vi "EOL Sunshade Servo Test.vi"(7 "scaling factor":dbl=11.1, 10 "input cluster":T2={"Application Status"="", "Switch Output Array"=[], "Switch Value Configuration"=[], "NVH Configuration"={"NVH Station?"=FALSE, "nvh app instance path"="", "NVH_ErrorMessages sv url"="", "NVH_Inputs sv url"="", "NVH_MotionNumber sv url"="", "NVH_Outputs sv url"="", "NVH_PartNumber sv url"="", "NVH_PartNumber_Echo sv url"="", "NVH_SerialNumber sv url"="", "NVH_AmbientTempF sv url"=""}, "rs232 port map"={"PMAC"="", "PS Port"="", "LVDT Unit"="", "RS232"=""}, "ethernet address map"={"LVDT 1 Unit"="172.17.53.143", "LVDT Unit 1 port"=0}, "paths"={"Base Path"=path "", "system error log path"=path "", "Error Table Path"=path "C/Labview Code/System/Error Table", "Store errors log path"=path "C/Labview Code/System/Error Table", "data bytes log path"=path "C/Labview Code/System/Error Table", "network path"=path "C/Labview Code/System/Error Table"}, "Station Index"=0, "Store Data"={"Motion Data Array"=[], "Error Table"=[], "Sun Shade Close Force Limits"={"Overall Min"=0.0, "Overall Max"=0.0, "Avg Min"=0.0, "Avg Max"=0.0, "Truncation Start"=0.0, "Truncation End"=0.0, "Variance"=0.0, "Check Noise"=FALSE}, "Sun Shade Open Force Limits"={"Overall Min"=0.0, "Overall Max"=0.0, "Avg Min"=0.0, "Avg Max"=0.0, "Truncation Start"=0.0, "Truncation End"=0.0, "Variance"=0.0, "Check Noise"=FALSE}, "Sunshade Open Data"=[], "Sunshade Close Data"=[], "Module Info"={"Serial Number"="", "Pallet Number"="", "Sunshade Color"="", "Inalfa Part Number"="", "Customer Number"=""}, "Sunsahde Close Raw Data"=[], "Sunshade Open Raw Data"=[], "Software Version"=[], "Constant Version"=[], "Hardware Version"=[], "Inalfa Part Number ECU"=[], "LVDT Data"=[], "Communication Line 1"=[], "Communication Line 2"=[], "Anti Pinch Force"=[], "Cycle Time"="", "Anti Pinch Vent Force"=[], "iGPS LVDT Data"=[], "data bytes log"=""}, "D in map"={"Abort Test"=enum."Dev2/port2/line6", "Start Test"=enum."Dev2/port2/line6"}, "DO Task"="", "ctl refs"={"Start Test"=refnum, "Abort Test"=refnum, "Manual Control"=refnum, "Route to Repair"=refnum, "Waveform Graph"=refnum, "Motion Data"=refnum, "all station status"=refnum, "Individual Station Status"=refnum, "exit program"=refnum, "Sunshade Servo Data Open"=refnum, "Sunshade Servo Data Close"=refnum, "Red-Rabbit Mode"=refnum, "Direct Manual Ctrl"=refnum}, "misc station config"={"Station Name"="", "is AT station?"=FALSE, "is audit station?"=FALSE, "power supply type"=enum."GENser", "use alt China TP2 LVDT Logic Seq"=FALSE, "hmi operator abort timeout"=0, "dump all analog values even if pass"=FALSE, "debug log pre-filter ap stream bytes"=FALSE, "use separate lvdt x and z extend tags"=FALSE, "is print"=FALSE}, "ethernet tcp refs"={"LVDT Unit"=refnum}, "Sunshade Barcode Scan"={"Sunshade Number 2"="", "Sunshade Number 1"="", "Keyence tuning bank idx"=0}, "AP Test Data"={"Raw Sunshade AP Data"="", "Raw Glass AP Data"="", "PMAC Read Counter"=0.0, "Database AP Data"=[]}, "Motion Status"={"hmi operator abort start time"=0, "Current Data Index"=0, "Analog Data"=[], "Motor Position Hex"=0, "Messages Index"=0, "Last Bytes"=[], "Current Hall Position"=0, "Motion Stop Timer"=0, "Position Test"=enum."Not Tested", "Noise Test"=enum."Not Tested", "motion stop check initialized"=FALSE, "remote sense enabled"=FALSE, "Motion"=enum."Glass Teach"}, "LVDT Status"={"LVDT's stored config"=[], "lvdt precision"={"truncate instead of rounding"=FALSE, "decimal places"=0}}, "Sequence State"={"Step Description"="", "Cycle Start Time"=0, "Step Data String"="", "Pass?"=FALSE, "Seqence"=[], "Active Step"=0, "Testing?"=FALSE, "Red-Rabbit Mode"=FALSE, "route-to-repair mode"=FALSE, "NVH Status"={"Restart IRQ Counter"=0, "NVH Test Needed?"=FALSE, "NVH Test Running?"=FALSE}, "Present (s)"=0.0, "Hold Mode?"=FALSE, "Hold?"=FALSE, "Rx Invalid?"=FALSE}, "misc status"={"delay start time (ticks)"=0, "In Vehicle Mode?"=FALSE, "Diag Mode?"=FALSE, "Serial Port Configured?"=FALSE, "PS Voltage"=0.0, "Diag Serial Port"="", "Part Setup"={"Communication Type"=enum."None", "Send Messages to"=enum."Glass", "RAP Signal"=enum."High", "Motor Type"=enum."Smart Motor", "NVH Part Number"=0, "Turn Off Timer"=0, "Part Type"=""}, "Part History Number"="", "Plant Number"=0, "AP Data Type"=enum."91/61", "Real Rollo?"=FALSE}, "NVH Operator?"=FALSE, "NVH Pass?"=FALSE, "Operator Pass?"=FALSE, "Operator Action?"=FALSE, "Noise Source"=0, "USBHandle"=0, "PeakInfo"="", "PeakNumber"=0, "NVH Motion Steps"=[], "Second Check?"=FALSE, "Decibel data"=[], "Direct Control Info"={"EnableStopOnHome"=FALSE, "EnableStopOnPos"=FALSE, "TeachEvent"=FALSE, "open offset"=0, "close offset"=0, "Derect control"=FALSE, "set position"=[], "teach pass "=FALSE, "Drift offsets"=[], "Hall Positions"=[]}, "manual control(direct)"=FALSE, "LIN INFO"={"Toolkit Type"=enum."Inalfa LIN", "NAD"=36, "Inalfa LIN"={"Master Frame(3C)"="", "Slave Frame(3D)"="NIXNET_exampleLDF", "Request Schedule"="NIXNET_exampleLDF", "Response Schedule"="CEMLIN3DiagResponseSchedule\nSPA3414_ConfigurationsCMAGeely_CEMCALYPSOSDB34XX0Cfg_LIN3_190709_", "Frame Write SCU"="", "Frame Read SCU"="", "LIN Name"=""}, "ADCS LIN"={"Port"="MasterReq\nSPA3414_ConfigurationsCMAGeely_CEMCALYPSOSDB34XX0Cfg_LIN3_190709_", "HW select"=0, "XNET Cluster"="SlaveResp\nSPA3414_ConfigurationsCMAGeely_CEMCALYPSOSDB34XX0Cfg_LIN3_190709_", "ByteCmd Path"=path "C/Labview Code/System/ByteCmdConfig.txt"}, "TS LIN"={"ref info"=refnum, "LIN Channel"=0, "ByteCmd Path"=path "C/Labview Code/System/ByteCmdConfig.txt"}}, "Config Info"=variant} {"LIN INFO"."NAD" format="%.0x"; "LIN INFO"."ADCS LIN"."HW select" items=["NI-XNET", "NI-CAN"]; "LVDT Status"."LVDT's stored config"."Lower Limit" format="%.2f"; "LVDT Status"."LVDT's stored config"."Upper Limit" format="%.2f"; "Store Data"."Sun Shade Open Force Limits"."Variance" format="%.2g"; "Store Data"."Sun Shade Open Force Limits"."Truncation End" format="%.2g"; "Store Data"."Sun Shade Open Force Limits"."Truncation Start" format="%.2g"; "Store Data"."Sun Shade Open Force Limits"."Avg Max" format="%.2g"; "Store Data"."Sun Shade Open Force Limits"."Avg Min" format="%.2g"; "Store Data"."Sun Shade Open Force Limits"."Overall Max" format="%.2g"; "Store Data"."Sun Shade Open Force Limits"."Overall Min" format="%.2g"; "Store Data"."Sun Shade Close Force Limits"."Variance" format="%.2g"; "Store Data"."Sun Shade Close Force Limits"."Truncation End" format="%.2g"; "Store Data"."Sun Shade Close Force Limits"."Truncation Start" format="%.2g"; "Store Data"."Sun Shade Close Force Limits"."Avg Max" format="%.2g"; "Store Data"."Sun Shade Close Force Limits"."Avg Min" format="%.2g"; "Store Data"."Sun Shade Close Force Limits"."Overall Max" format="%.2g"; "Store Data"."Sun Shade Close Force Limits"."Overall Min" format="%.2g"; "Store Data"."Motion Data Array"."Motion Data Limits"."LIN Msg"."Msg" format="%02x"; "Store Data"."Motion Data Array"."Motion Data Limits"."LIN Msg"."ID" format="%02x"}, 11 "Sunshade Close Test?":bool) -> (0 "Error Table Out":string[][](array[string]), 1 "Sunshade Raw Data":dbl[](graph), 2 "Sunshade Calculated Data":dbl[](array[numeric]), 3 "Pass? Out":bool, 5 "ss servo limits":T1 {"Variance" format="%.2g"; "Truncation End" format="%.2g"; "Truncation Start" format="%.2g"; "Avg Max" format="%.2g"; "Avg Min" format="%.2g"; "Overall Max" format="%.2g"; "Overall Min" format="%.2g"})   [LabVIEW 2018]
uses:
  02.Type Def's/main state cluster.ctl
  02.Type Def's/All Switch Configuration Cluster.ctl
  02.Type Def's/All Motions.ctl
  02.Type Def's/EOL Switch Value Configuration Cluster.ctl
  02.Type Def's/EOL Switch Max Min Check Cluster.ctl
  02.Type Def's/station nvh config.ctl
  02.Type Def's/station rs232 port map.ctl
  02.Type Def's/station ethernet address map.ctl
  02.Type Def's/station paths.ctl
  02.Type Def's/EOL Save Module Test Data Control.ctl
  02.Type Def's/EOL Motion Database Table.ctl
  05.UserVI's/type defs/17x Audit Motion Data Seq Control.ctl
  05.UserVI's/type defs/17x AP Data Type.ctl
  05.UserVI's/type defs/17x Sunshade Limts Seq.ctl
  02.Type Def's/EOL Module Info Control.ctl
  02.Type Def's/station DI map.ctl
  05.UserVI's/type defs/EOL Global Digital Input Control.ctl
  02.Type Def's/control refs.ctl
  02.Type Def's/station motion data indicator.ctl
  02.Type Def's/Screen Motion Data.ctl
  02.Type Def's/Pass Fail Control.ctl
  02.Type Def's/station hmi.ctl
  02.Type Def's/lvdt name val pair.ctl
  02.Type Def's/individual station status.ctl
  02.Type Def's/misc station config.ctl
  05.UserVI's/Lambda Power/power supply types.ctl
  05.UserVI's/type defs/EOL LVDT's Check Controller.ctl
  05.UserVI's/LVDT's/lvdt precision.ctl
  02.Type Def's/sequence state.ctl
  05.UserVI's/sequence/type defs/Sequence Info.ctl
  05.UserVI's/type defs/EOL Part Setup.ctl
  02.Type Def's/All Communication Types.ctl
  05.UserVI's/type defs/Communication with Motors.ctl
  05.UserVI's/type defs/RAP Signal Control.ctl
  05.UserVI's/type defs/EOL Motor Type.ctl
  02.Type Def's/station LIN config.ctl
  03.Inalfa LIN/LIN Device.ctl
  <vilib>/CMC.AME/Inalfa ADCS/Ctl'Def/ADCS_LIN info.ctl
  C:/Program Files (x86)/National Instruments/LabVIEW 2018/vi.lib/CMC.AME/Inalfa TS LIN/TOSUN/TSMaster/bin/Interop.TSMasterAPI.dll
  Program Files (x86)/National Instruments/LabVIEW 2018/vi.lib/CMC.AME/Inalfa TS LIN/TOSUN/TSMaster/bin/Interop.TSMasterAPI.dll
  06.Test Loop/Sub'VIs/Type Def's/Config Info.ctl
  02.Type Def's/EOL Analog Input Control.ctl
  02.Type Def's/NVH Digital Input.ctl
  02.Type Def's/NVH Mode Control 2.0.ctl
  02.Type Def's/NVH Digital Output.ctl
panel:
  out "Cleared data":dbl[][](array[numeric])
  out "Current Out New":dbl[](graph)
  out "Current Out":dbl[](graph)
  out "State":string
  # "Min"
  # "N"
  # "Min"
  # "Start"
  # "N"
  # "Max"
  # "N"
  # "Max"
  # "N"
  # "End"
  # "Sunroof Barcode"
  # "Pallet Number"
  # "Part Type"
  # "Application Status"
  # "Current Step"
  # "Cycle Time"
  # "Pass / Fail"
  # "Shade Close"
  # "Actual Data"
  # "Limits"
  # "Avg Current"
  # "Run Time"
  # "Speed"
  # "Noise Test"
  # "Position"
  # "Shade Open"
  # "Actual Data"
  # "Limits"
  # "Avg Current"
  # "Run Time"
  # "Speed"
  # "Noise Test"
  # "Position"
  # "Vent Close"
  # "Actual Data"
  # "Limits"
  # "Avg Current"
  # "Run Time"
  # "Speed"
  # "Noise Test"
  # "Position"
  # "Vent Open"
  # "Actual Data"
  # "Limits"
  # "Avg Current"
  # "Run Time"
  # "Speed"
  # "Noise Test"
  # "Position"
  # "Slide Close"
  # "Actual Data"
  # "Limits"
  # "Avg Current"
  # "Run Time"
  # "Speed"
  # "Noise Test"
  # "Position"
  # "Slide Open"
  # "Actual Data"
  # "Limits"
  # "Avg Current"
  # "Run Time"
  # "Speed"
  # "Noise Test"
  # "Position"
  # "Min"
  # "N"
  # "Min"
  # "Start"
  # "N"
  # "Max"
  # "N"
  # "Max"
  # "N"
  # "End"
  # "Min"
  # "N"
  # "Min"
  # "Start"
  # "N"
  # "Max"
  # "N"
  # "Max"
  # "N"
  # "End"
  # "Min"
  # "Max"
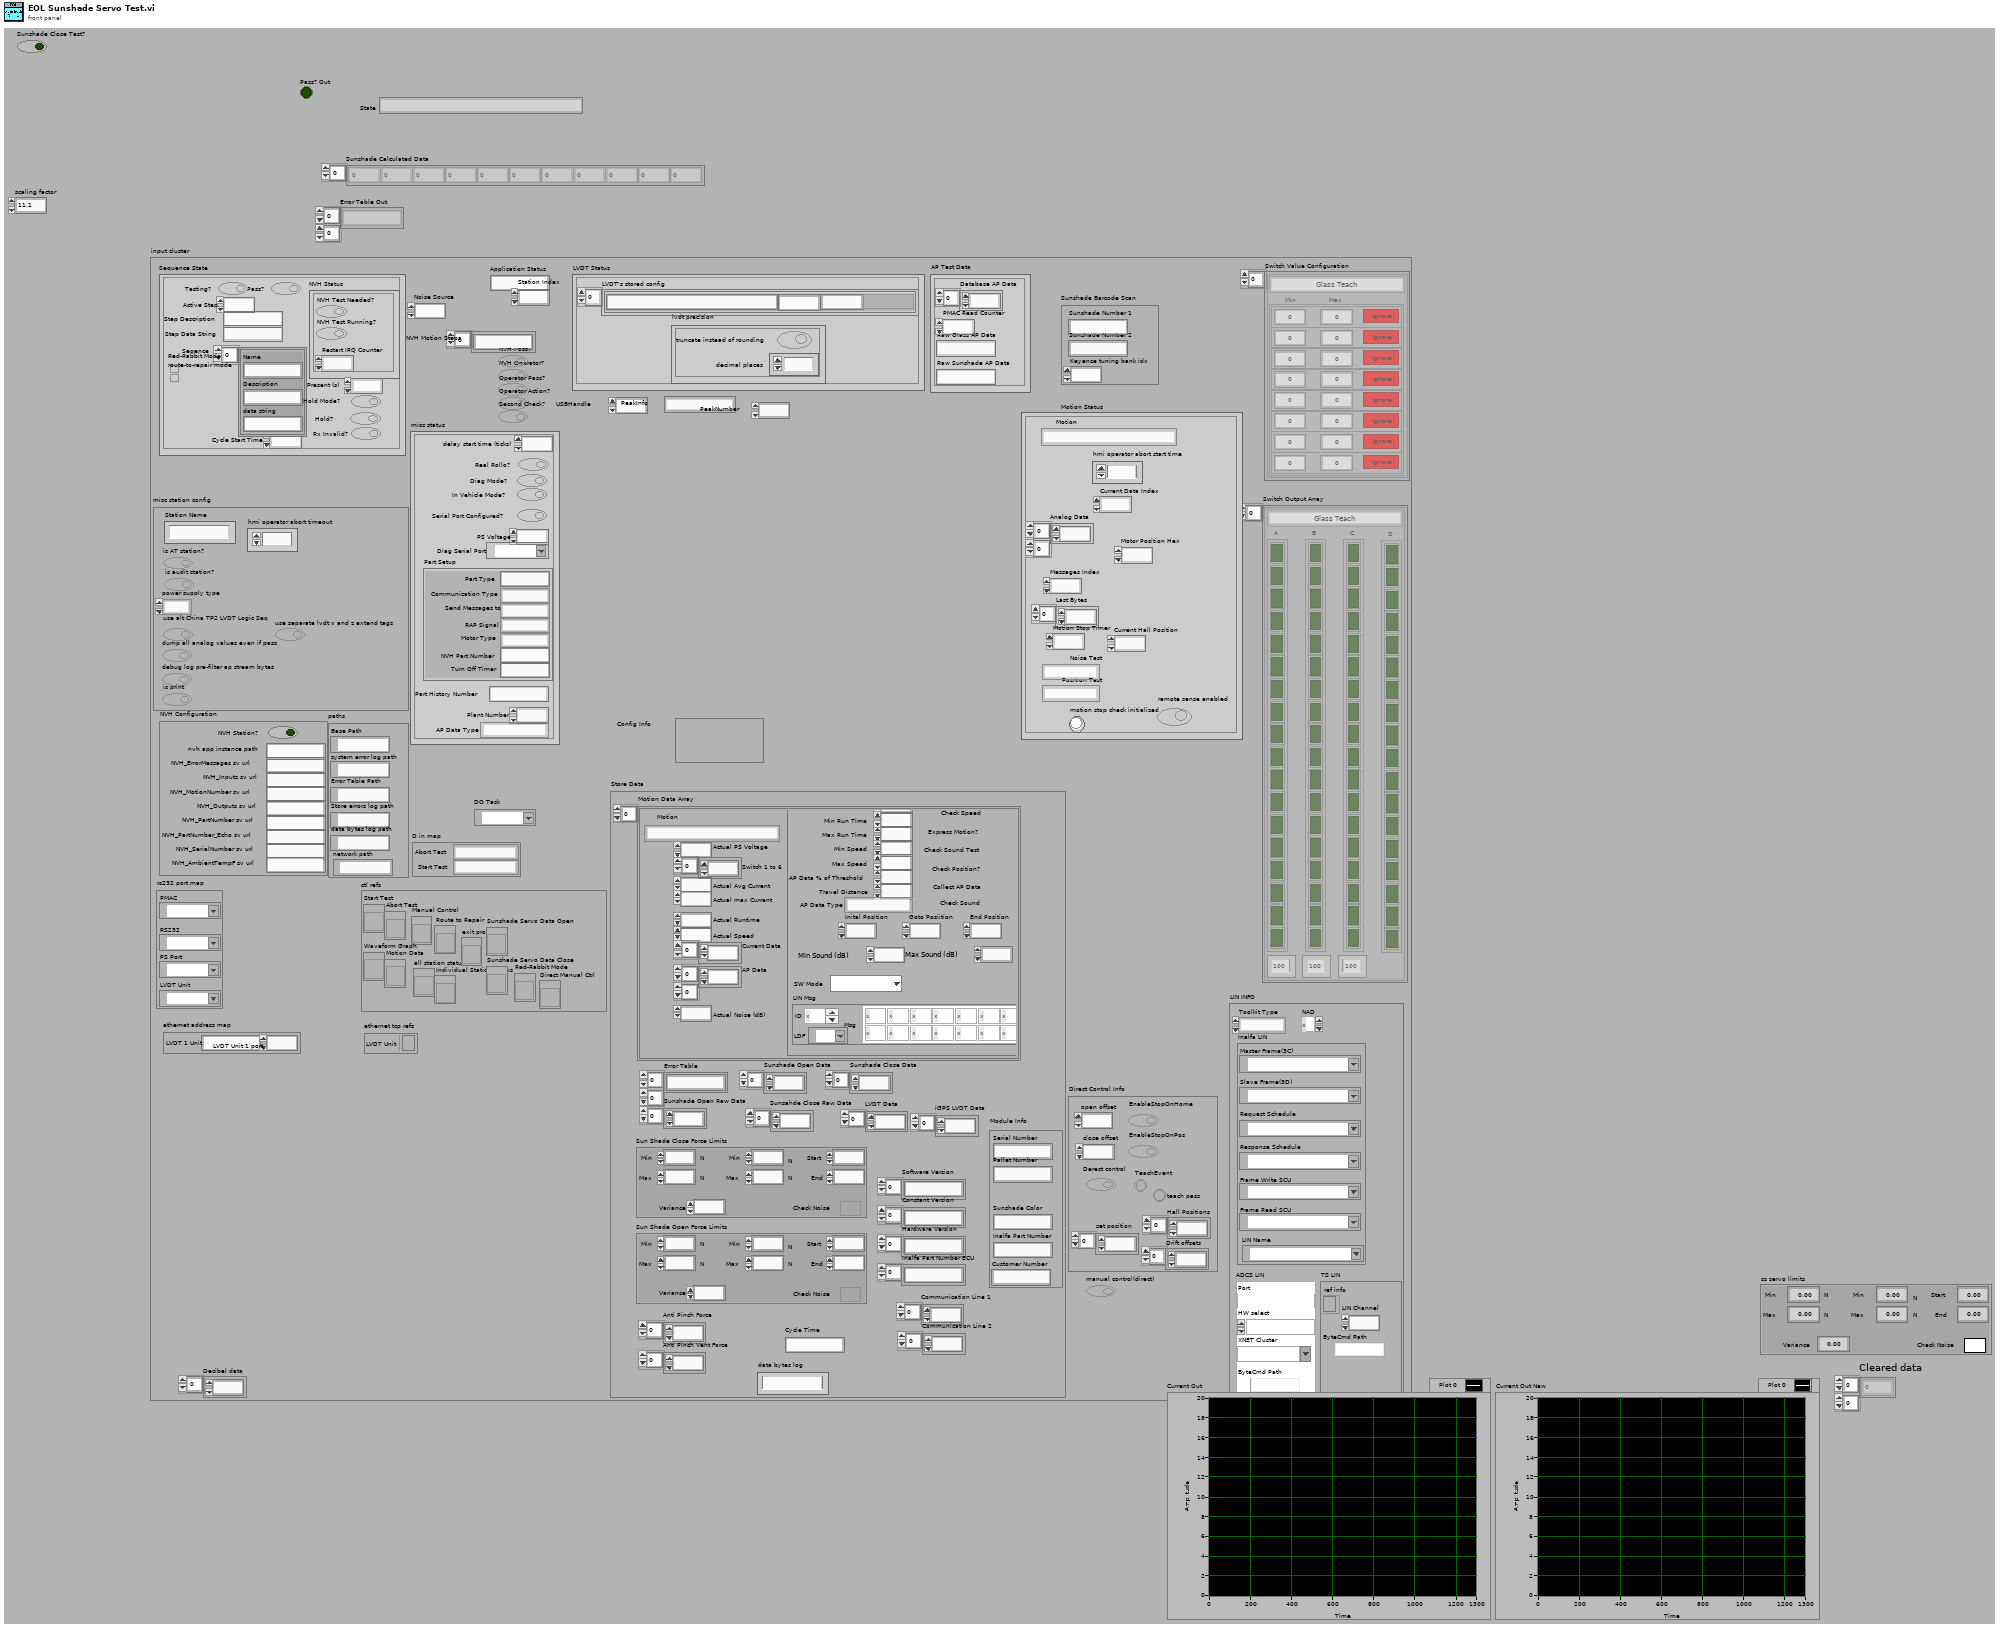
[diagram p1: front panel]
types:
  T1 = typedef "17x Sunshade Limts Seq.ctl" = cluster{"Overall Min":dbl, "Overall Max":dbl, "Avg Min":dbl, "Avg Max":dbl, "Truncation Start":dbl, "Truncation End":dbl, "Variance":dbl, "Check Noise":bool}
  T2 = typedef "main state cluster.ctl" = cluster{"Application Status":string, "Switch Output Array":T3[], "Switch Value Configuration":T5[], "NVH Configuration":T7, "rs232 port map":T8, "ethernet address map":T9, "paths":T10, "Station Index":i32, "Store Data":T11, "D in map":T16, "DO Task":refnum<k21>, "ctl refs":T18, "misc station config":T19, "ethernet tcp refs":cluster{"LVDT Unit":refnum<k5>}, "Sunshade Barcode Scan":cluster{"Sunshade Number 2":string, "Sunshade Number 1":string, "Keyence tuning bank idx":i32}, "AP Test Data":cluster{"Raw Sunshade AP Data":string, "Raw Glass AP Data":string, "PMAC Read Counter":dbl, "Database AP Data":dbl[]}, "Motion Status":cluster{"hmi operator abort start time":u32, "Current Data Index":i32, "Analog Data":sgl[][], "Motor Position Hex":u16, "Messages Index":u16, "Last Bytes":u8[], "Current Hall Position":i16, "Motion Stop Timer":u32, "Position Test":T21, "Noise Test":T21, "motion stop check initialized":bool, "remote sense enabled":bool, "Motion":T4}, "LVDT Status":cluster{"LVDT's stored config":T22[], "lvdt precision":T23}, "Sequence State":T24, "misc status":cluster{"delay start time (ticks)":u32, "In Vehicle Mode?":bool, "Diag Mode?":bool, "Serial Port Configured?":bool, "PS Voltage":dbl, "Diag Serial Port":refnum<visa-resource-name>, "Part Setup":T26, "Part History Number":string, "Plant Number":u8, "AP Data Type":T14, "Real Rollo?":bool}, "NVH Operator?":bool, "NVH Pass?":bool, "Operator Pass?":bool, "Operator Action?":bool, "Noise Source":u32, "USBHandle":i32, "PeakInfo":string, "PeakNumber":i32, "NVH Motion Steps":string[], "Second Check?":bool, "Decibel data":dbl[], "Direct Control Info":cluster{"EnableStopOnHome":bool, "EnableStopOnPos":bool, "TeachEvent":bool, "open offset":i32, "close offset":i32, "Derect control":bool, "set position":i32[], "teach pass ":bool, "Drift offsets":i32[], "Hall Positions":i32[]}, "manual control(direct)":bool, "LIN INFO":T31, "Config Info":T34}
  T3 = typedef "All Switch Configuration Cluster.ctl" = cluster{"All Motions":T4, "A":bool[], "B":bool[], "C":bool[], "D":bool[], "A activation time (ms)":u32, "B activation time (ms)":u32, "C activation time (ms)":u32}
  T4 = typedef "All Motions.ctl" = enum16{"Glass Teach", "Glass Slide Open", "Glass Slide Close", "Glass Vent Open", "Glass Vent Close", "Sunshade Teach", "Sunshade Open", "Sunshade Close", "Idle", "Sunshade Open 2", "Sunshade Close 2", "Glass Slide Open Sunshade Open", "Glass Slide Open Sunshade Close", "Glass Slide Close Sunshade Open", "Glass Slide Close Sunshade Close", "Glass Vent Open Sunshade Open", "Glass Vent Open Sunshade Close", "Glass Vent Close Sunshade Open", "Glass Vent Close Sunshade Close", "Express Glass Slide Open", "Express Glass Slide Close", "Express Glass Vent Open", "Express Glass Vent Close", "Express Sunshade Open", "Express Sunshade Close", "Express Sunshade Open 2", "Express Sunshade Close 2", "Express Glass Slide Open Sunshade Open", "Express Glass Slide Open Sunshade Close", "Express Glass Slide Close Sunshade Open", "Express Glass Slide Close Sunshade Close", "Express Glass Vent Open Sunshade Open", "Express Glass Vent Open Sunshade Close", "Express Glass Vent Close Sunshade Open", "Express Glass Vent Close Sunshade Close", "Goto Position Glass", "Goto Position Sunshade", "Sunshade Teach 2"}
  T5 = typedef "EOL Switch Value Configuration Cluster.ctl" = cluster{"All Motions":T4, "Array":T6[]}
  T6 = typedef "EOL Switch Max Min Check Cluster.ctl" = cluster{"Min":dbl, "Max":dbl, "Check?":bool}
  T7 = typedef "station nvh config.ctl" = cluster{"NVH Station?":bool, "nvh app instance path":string, "NVH_ErrorMessages sv url":string, "NVH_Inputs sv url":string, "NVH_MotionNumber sv url":string, "NVH_Outputs sv url":string, "NVH_PartNumber sv url":string, "NVH_PartNumber_Echo sv url":string, "NVH_SerialNumber sv url":string, "NVH_AmbientTempF sv url":string}
  T8 = typedef "station rs232 port map.ctl" = cluster{"PMAC":refnum<visa-resource-name>, "PS Port":refnum<visa-resource-name>, "LVDT Unit":refnum<visa-resource-name>, "RS232":refnum<visa-resource-name>}
  T9 = typedef "station ethernet address map.ctl" = cluster{"LVDT 1 Unit":string, "LVDT Unit 1 port":u16}
  T10 = typedef "station paths.ctl" = cluster{"Base Path":path, "system error log path":path, "Error Table Path":path, "Store errors log path":path, "data bytes log path":path, "network path":path}
  T11 = typedef "EOL Save Module Test Data Control.ctl" = cluster{"Motion Data Array":T12[], "Error Table":string[][], "Sun Shade Close Force Limits":T1, "Sun Shade Open Force Limits":T1, "Sunshade Open Data":sgl[], "Sunshade Close Data":sgl[], "Module Info":T15, "Sunsahde Close Raw Data":sgl[], "Sunshade Open Raw Data":sgl[], "Software Version":string[], "Constant Version":string[], "Hardware Version":string[], "Inalfa Part Number ECU":string[], "LVDT Data":sgl[], "Communication Line 1":sgl[], "Communication Line 2":sgl[], "Anti Pinch Force":sgl[], "Cycle Time":string, "Anti Pinch Vent Force":sgl[], "iGPS LVDT Data":sgl[], "data bytes log":string}
  T12 = typedef "EOL Motion Database Table.ctl" = cluster{"Motion":T4, "Actual Avg Current":dbl, "Actual Runtime":dbl, "Actual Speed":dbl, "Current Data":sgl[], "Motion Data Limits":T13, "Switch 1 to 6":dbl[], "Actual PS Voltage":dbl, "AP Data":i16[][], "Actual max Current":dbl, "Actual Noise (dB)":dbl}
  T13 = typedef "17x Audit Motion Data Seq Control.ctl" = cluster{"Power Supply Voltage":dbl, "Min Avg Current":dbl, "Max Avg Current":dbl, "Min Run Time":dbl, "Max Run Time":dbl, "Min Speed":dbl, "Max Speed":dbl, "AP Data % of Threshold":dbl, "Travel Distance":dbl, "AP Data Type":T14, "Check Current":bool, "Check Run Time":bool, "Check Speed":bool, "Express Motion?":bool, "Check Sound Test":bool, "Check Position?":bool, "Collect AP Data":bool, "Inital Position":u16, "End Position":u16, "Goto Posiition":u16, "Max max Current":dbl, "Min max Current":dbl, "Check max Current":bool, "Check Sound":bool, "Min Sound (dB)":dbl, "Max Sound (dB)":dbl, "SW Mode":enum16{"Hard Switch", "Uncond Frame"}, "LIN Msg":cluster{"ID":u8, "Msg":u8[][], "LDF":refnum<k21>}}
  T14 = typedef "17x AP Data Type.ctl" = enum16{"91/61", "92/62", "93/63", "67", "68", "6F", "71", "91 Msg", "92 Msg", "93 Msg", "94 Msg", "HiRain 91", "HiRain 92 Speed", "HiRain 92 HS", "HiRain 92", "HiRain 93", "SnT"}
  T15 = typedef "EOL Module Info Control.ctl" = cluster{"Serial Number":string, "Pallet Number":string, "Sunshade Color":string, "Inalfa Part Number":string, "Customer Number":string}
  T16 = typedef "station DI map.ctl" = cluster{"Abort Test":T17, "Start Test":T17}
  T17 = typedef "EOL Global Digital Input Control.ctl" = enum16{"Dev2/port0/line0", "Dev2/port0/line1", "Dev2/port0/line2", "Dev2/port0/line3", "Dev2/port0/line4", "Dev2/port0/line5", "Dev2/port0/line6", "Dev2/port0/line7", "Dev2/port1/line0", "Dev2/port1/line1", "Dev2/port1/line2", "Dev2/port1/line3", "Dev2/port1/line4", "Dev2/port1/line5", "Dev2/port1/line6", "Dev2/port1/line7", "Dev2/port2/line0", "Dev2/port2/line1", "Dev2/port2/line2", "Dev2/port2/line3", "Dev2/port2/line4", "Dev2/port2/line5", "Dev2/port2/line6", "Dev2/port2/line7", "Prerun Start Test", "Prerun Abort Test", "Audit Start Test", "Audit Abort Test", "Dev2/port3/line4", "Dev2/port3/line5", "Breakin Start Test", "Breakin Abort Test", "Not Implemented"}
  T18 = typedef "control refs.ctl" = cluster{"Start Test":refnum<vi>, "Abort Test":refnum<vi>, "Manual Control":refnum<vi>, "Route to Repair":refnum<vi>, "Waveform Graph":refnum<vi>, "Motion Data":refnum<vi>, "all station status":refnum<vi>, "Individual Station Status":refnum<vi>, "exit program":refnum<vi>, "Sunshade Servo Data Open":refnum<vi>, "Sunshade Servo Data Close":refnum<vi>, "Red-Rabbit Mode":refnum<vi>, "Direct Manual Ctrl":refnum<vi>}
  T19 = typedef "misc station config.ctl" = cluster{"Station Name":string, "is AT station?":bool, "is audit station?":bool, "power supply type":T20, "use alt China TP2 LVDT Logic Seq":bool, "hmi operator abort timeout":u32, "dump all analog values even if pass":bool, "debug log pre-filter ap stream bytes":bool, "use separate lvdt x and z extend tags":bool, "is print":bool}
  T20 = typedef "power supply types.ctl" = enum16{"GENser", "ZUPser", "GENeth", "Manual", "ITECH"}
  T21 = typedef "Pass Fail Control.ctl" = enum16{"Not Tested", "Pass", "Fail"}
  T22 = typedef "EOL LVDT's Check Controller.ctl" = cluster{"Upper Limit":dbl, "Lower Limit":dbl, "LVDT Name":string, "Check":bool}
  T23 = typedef "lvdt precision.ctl" = cluster{"truncate instead of rounding":bool, "decimal places":u8}
  T24 = typedef "sequence state.ctl" = cluster{"Step Description":string, "Cycle Start Time":u32, "Step Data String":string, "Pass?":bool, "Seqence":T25[], "Active Step":u8, "Testing?":bool, "Red-Rabbit Mode":bool, "route-to-repair mode":bool, "NVH Status":cluster{"Restart IRQ Counter":u8, "NVH Test Needed?":bool, "NVH Test Running?":bool}, "Present (s)":dbl, "Hold Mode?":bool, "Hold?":bool, "Rx Invalid?":bool}
  T25 = typedef "Sequence Info.ctl" = cluster{"Name":string, "Description":string, "data string":string}
  T26 = typedef "EOL Part Setup.ctl" = cluster{"Communication Type":T27, "Send Messages to":T28, "RAP Signal":T29, "Motor Type":T30, "NVH Part Number":u16, "Turn Off Timer":u16, "Part Type":string}
  T27 = typedef "All Communication Types.ctl" = enum16{"None", "CAN", "RS 232", "RS 232 LIN", "GM LIN", "SnT LIN", "K Line", "Robel CAN", "P42M-Continental", "Inalfa SCU LIN", "Spare 3"}
  T28 = typedef "Communication with Motors.ctl" = enum16{"Glass", "Rollo", "Both"}
  T29 = typedef "RAP Signal Control.ctl" = enum16{"High", "Low", "None"}
  T30 = typedef "EOL Motor Type.ctl" = enum16{"Smart Motor", "Sensor Motor"}
  T31 = typedef "station LIN config.ctl" = cluster{"Toolkit Type":enum16{"Inalfa LIN", "ADCS LIN", "TS LIN"}, "NAD":u8, "Inalfa LIN":T32, "ADCS LIN":T33, "TS LIN":cluster{"ref info":refnum<k24>, "LIN Channel":i32, "ByteCmd Path":path}}
  T32 = typedef "LIN Device.ctl" = cluster{"Master Frame(3C)":refnum<k21>, "Slave Frame(3D)":refnum<k21>, "Request Schedule":refnum<k21>, "Response Schedule":refnum<k21>, "Frame Write SCU":refnum<k21>, "Frame Read SCU":refnum<k21>, "LIN Name":refnum<k21>}
  T33 = typedef "ADCS_LIN info.ctl" = cluster{"Port":string, "HW select":u16, "XNET Cluster":string, "ByteCmd Path":path}
  T34 = typedef "Config Info.ctl" = variant
  T35 = typedef "plc comms params.ctl" = cluster{"PLC boolean read Tags":T36, "PLC bool write Tags":T39, "PLC string read Tags":T40, "PLC string write Tags":T41, "use opc":bool, "PLC/OPC Path":string}
  T36 = typedef "station plc read boolean tags.ctl" = cluster{"AT glass position":T37, "AT shade position":T37, "AT in glass wand lower pos":T37, "AT in glass wand up pos":T37, "AT in sunshad wand lower pos":T37, "AT in sunshad wand up pos":T37, "AT in wand home pos":T37, "LVDT's Extended":T37, "bolt check 1":T37, "bolt check 2":T37, "bolt check 3":T37, "bolt check 4":T37, "bolt check 5":T37, "bolt check 6":T37, "bolt check 7":T37, "bolt check 8":T37, "start":T37, "abort":T37, "LVDT's Retracted":T37, "manual barcode print":T37, "ss servo at open":T37, "ss servo at close":T37, "ss servo opening":T37, "ss servo closing":T37, "control slide at home":T37, "control slide left good":T37, "control slide left over stroke":T37, "control slide right good":T37, "control slide right over stroke":T37, "wind deflector high speed pos":T37, "wind deflector low speed pos":T37, "AT VentPMACatHome":T37, "AT VentPMACisExtend":T37, "SS Barcode Scanner Bypassed":T37, "Check Frame Barcode":T37, "Z LVDTs Extended":T37, "NVH Operator Pass":T37, "NVH Operator Fail":T37, "NVH Operator Express Glass Open":T37, "NVH Operator Express Glass Close":T37, "NVH Operator Express Rollo Open01":T37, "NVH Operator Express Rollo Close01":T37, "NVH Operator Express Rollo Open02":T37, "NVH Operator Express Rollo Close02":T37, "NVH Operator Vent Open Noise":T37, "NVH Operator Vent Close Noise":T37, "NVH Operator Sunshade Open Noise":T37, "NVH Operator Sunshade Close Noise":T37, "NVH Operator Glass Open Noise":T37, "NVH Operator Glass Close Noise":T37, "NVH Operator Finish":T37, "NVH Operator Check":T37, "windproof position":T37, "NVH Operator Express Glass vent Open":T37, "NVH Operator Express Glass Vent Close":T37, "NVH Operator Re-do":T37, "AT at vent ATS test pos":T37, "AT at vent ATS Home pos":T37, "Start Adjust LVDT":T37, "Finish Adjust LVDT":T37}
  T37 = typedef "plc path and tag.ctl" = cluster{"Tag Name":string, "Network Path":string, "use opc":bool, "DataSocket Reference":T38}
  T38 = typedef "DataSocket Reference Type.ctl" = cluster{"CWDSLib._DCWDataSocket":refnum<k7>, "CWDSLib._DCWData":refnum<k7>, "OnDataUpdated":u32, "OnStatusUpdated":u32}
  T39 = typedef "station plc write boolean tags.ctl" = cluster{"AT set glass wand lower":T37, "AT set sunshade wand lower":T37, "AT set sunshade wand up":T37, "AT set glass wand up":T37, "AT set wand home pos":T37, "Test Complete Pass":T37, "Test Complete Fail":T37, "Test Started":T37, "Retract LVDT's":T37, "Extend LVDT's":T37, "ss servo open":T37, "ss servo close":T37, "control slide start":T37, "control slide stop":T37, "AT VentPMACHome":T37, "AT VentPMACExtended":T37, "Good Frame Barcode":T37, "Bad Frame Barcode":T37, "Extend Z LVDTS":T37, "NVH SunRoof Moving":T37, "NVH SunRoof Stop":T37, "NVH Pass":T37, "NVH Fail":T37, "NVH Operator Express Glass Opened":T37, "NVH Operator Express Glass Closed":T37, "NVH Operator Express Rollo Opened01":T37, "NVH Operator Express Rollo Closed01":T37, "NVH Operator Express Rollo Opened02":T37, "NVH Operator Pass":T37, "NVH Operator Fail":T37, "NVH Operator Check":T37, "NVH Operator Vent Open Noise":T37, "NVH Operator Vent Close Noise":T37, "NVH Operator Sunshade Open Noise":T37, "NVH Operator Sunshade Close Noise":T37, "NVH Operator Glass Open Noise":T37, "NVH Operator Glass Close Noise":T37, "NVH Operator Finish":T37, "Barcode01 OK":T37, "Barcode02 OK":T37, "AT set to Vent ATS Test Pos":T37, "AT set to Vent ATS Home Pos":T37, "Move LVDT Adjust Station":T37}
  T40 = typedef "station plc read string tags.ctl" = cluster{"Serial Number":T37, "Pallet Number":T37, "Inalfa Part Number":T37, "Shade Color":T37, "Model Type":T37, "Customer Number":T37, "Part History Number":T37, "Shade 1 Barcode":T37, "Shade 2 Barcode":T37, "Manual Serial Number":T37, "Manual Inalfa Part Number":T37, "Manual Shade Color":T37, "Manual Model Type":T37, "Manual Customer Number":T37, "Manual Part History Number":T37}
  T41 = typedef "station plc write string tags.ctl" = cluster{"barcode station error":T37, "error message 0":T37, "error message 1":T37, "error message 2":T37, "error message 3":T37}
  T42 = cluster{"Sunshade Raw Data":dbl[], "Sun Shade Close Force":T1, "Pass?":bool, "Error Table":string[][], "Sunshade Timer 2":dbl, "NVH Test Needed?":bool, "Sunshade Close Test?":bool, "NVH Noise Test OK?":bool, "Sunshade Calculated Data":dbl[], "Sunshade Timer 1":dbl, "Station Index":i32, "PLC boolean read Tags":T36, "PLC bool write Tags":T39, "NVH Configuration":T7}
  T43 = typedef "EOL Analog Input Control.ctl" = enum16{"SW PS  Volage", "Switch A", "Switch B", "Switch C", "Motor Voltage", "Motor Current", "ATS"}
  T44 = typedef "NVH Mode Control 2.0.ctl" = enum16{"Init", "Write", "Write String", "Read", "Write Part Number", "Write Motion Number", "Write Ambient TempF"}
  T45 = typedef "NVH Digital Input.ctl" = enum16{"Online", "Pass", "Fail", "Testing", "Ready for Model", "Error Bit 1", "Error Bit 2", "Error Bit 3", "Failure Bit 1", "Failure Bit 2", "Failure Bit 3", "Failure Bit 4", "Echo Bit 1", "Echo Bit 2", "Echo Bit 3", "Echo Bit 4", "Serial Number Read Ok", "Ready for Serrial Number"}
  T46 = typedef "NVH Digital Output.ctl" = enum16{"Restart IRQ", "Abort Test IRQ", "Read Model", "Start Test", "Stop Test", "End of Test IRQ", "Test Bit 1", "Test Bit 2", "Test Bit 3", "Test Bit 4", "Model Bit 1", "Model Bit 2", "Model Bit 3", "Model Bit 4", "Manual Restart IRQ"}
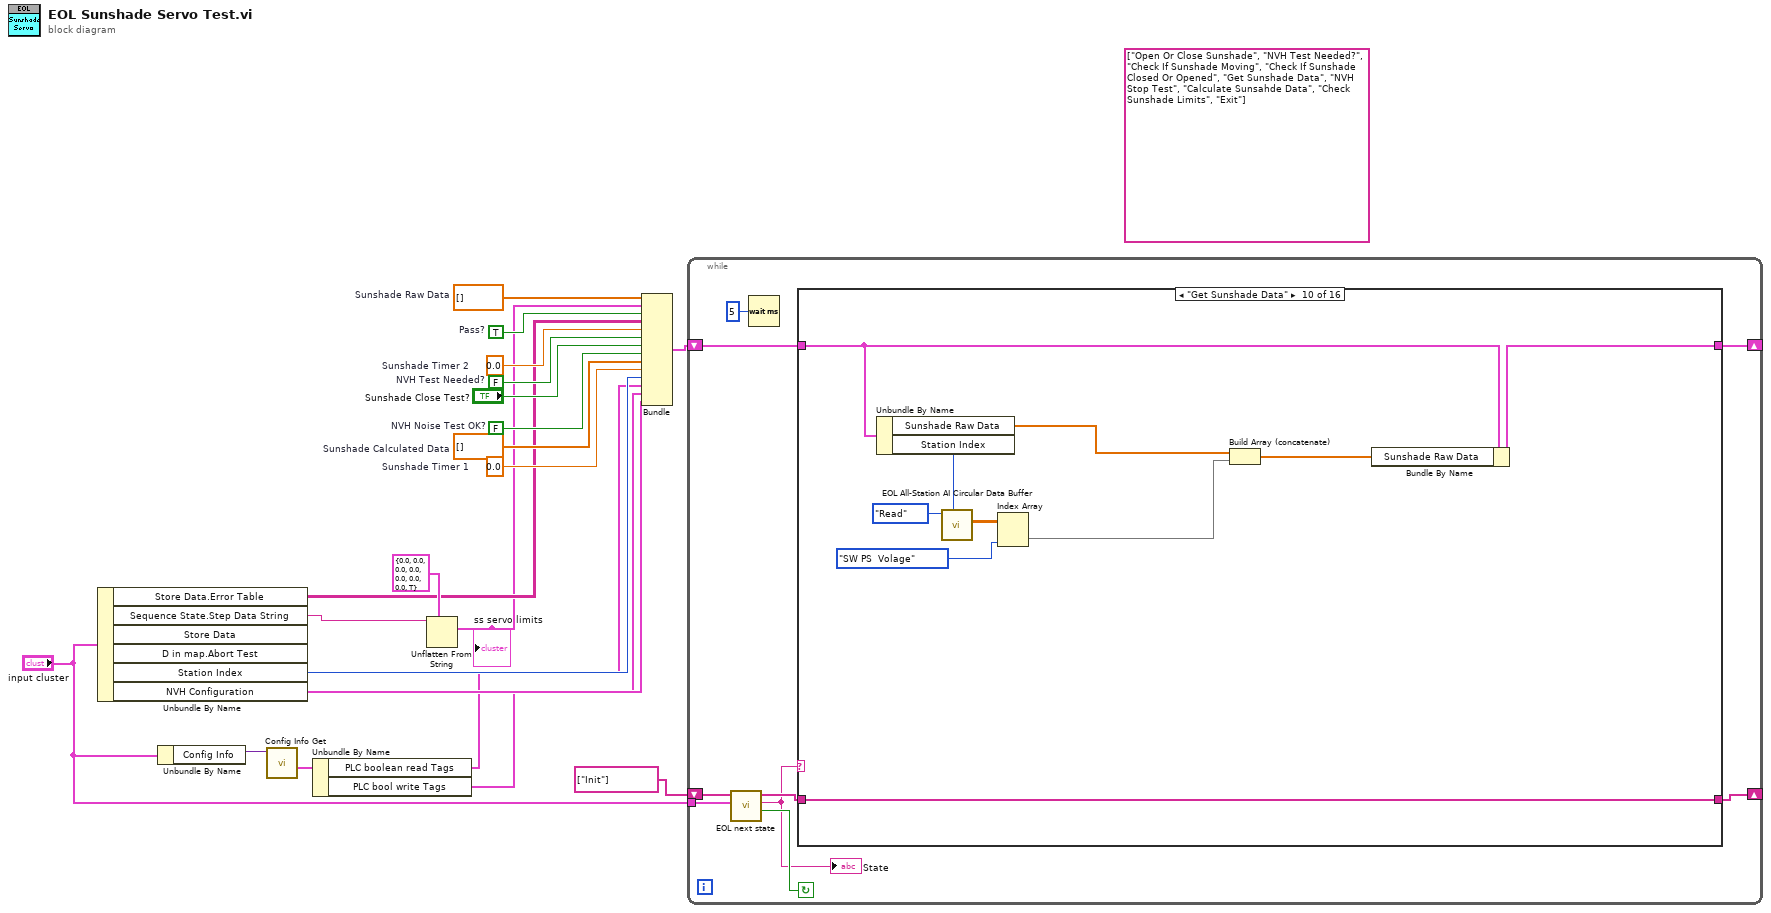
[diagram p0: block diagram]
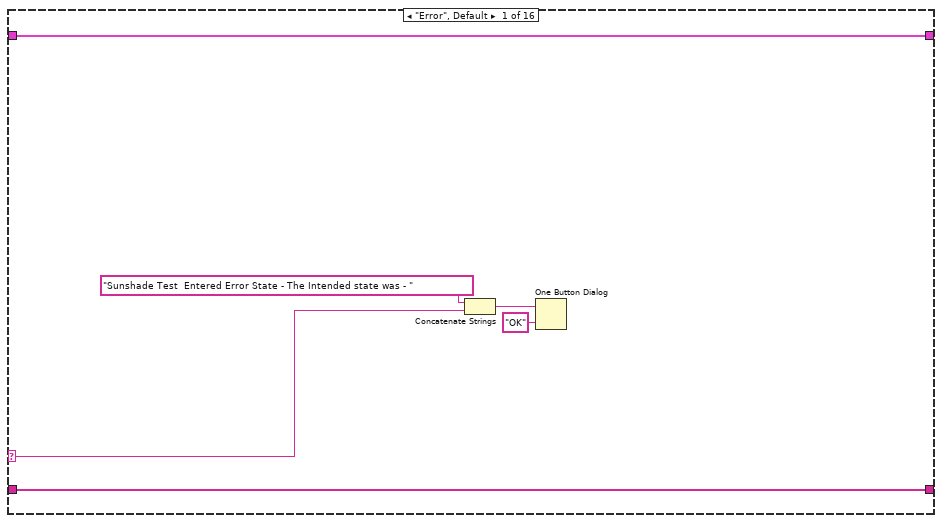
[diagram p2: hidden frame]
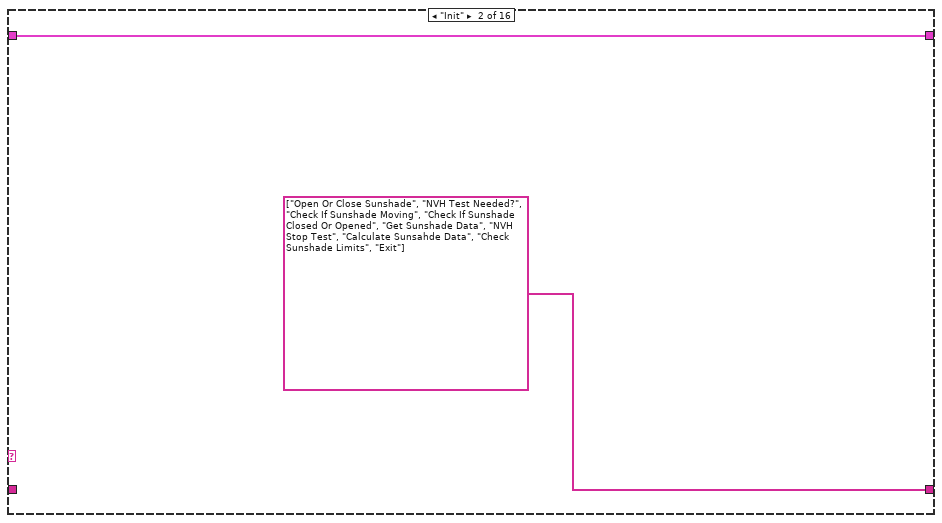
[diagram p3: hidden frame]
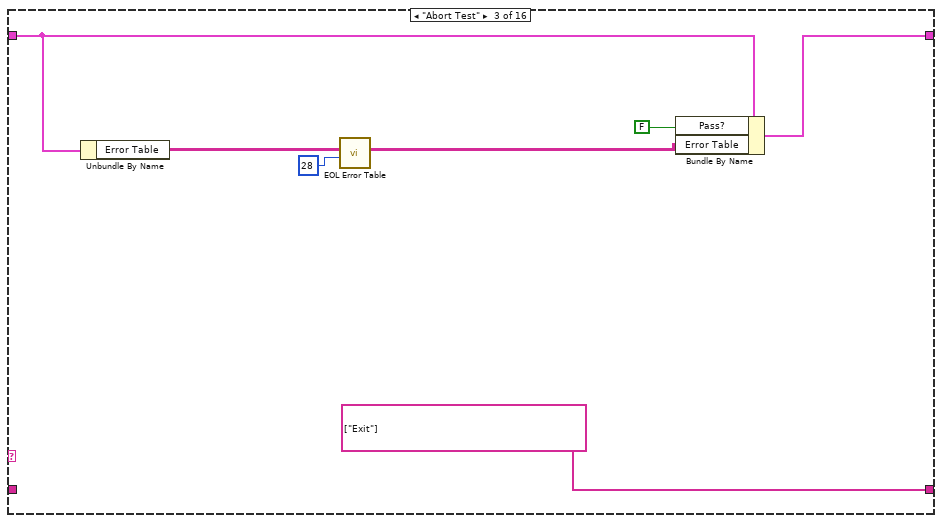
[diagram p4: hidden frame]
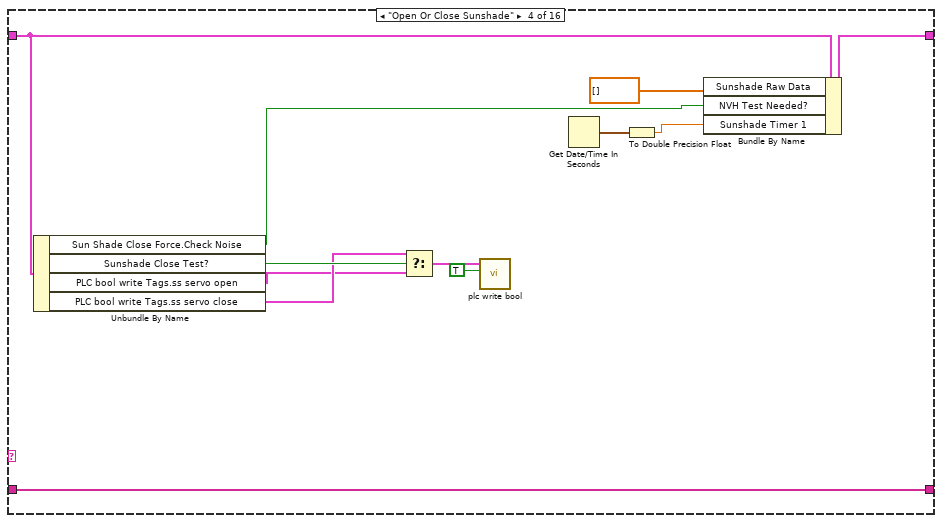
[diagram p5: hidden frame]
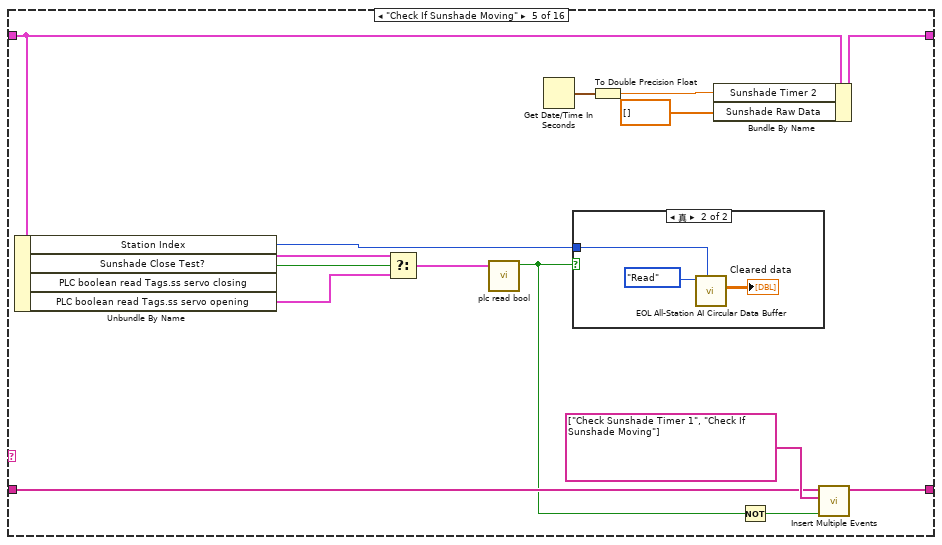
[diagram p6: hidden frame]
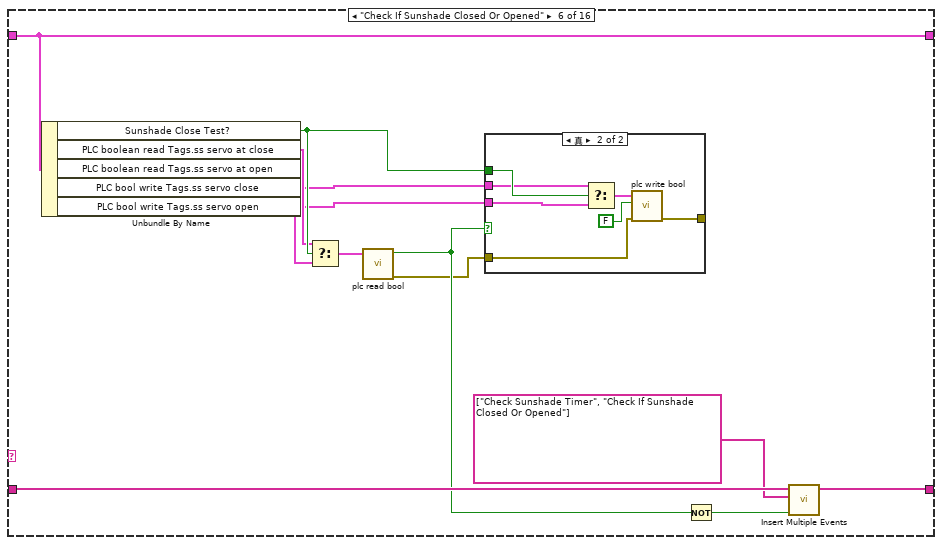
[diagram p8: hidden frame]
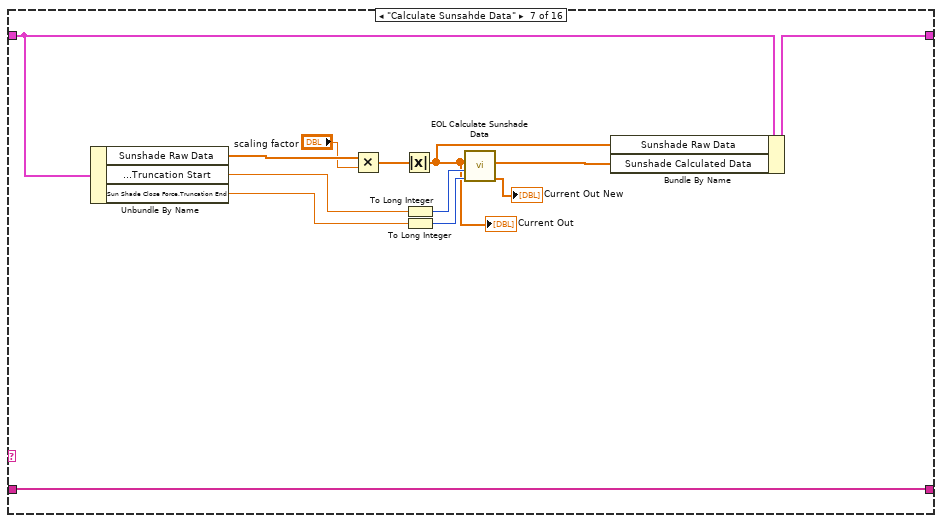
[diagram p10: hidden frame]
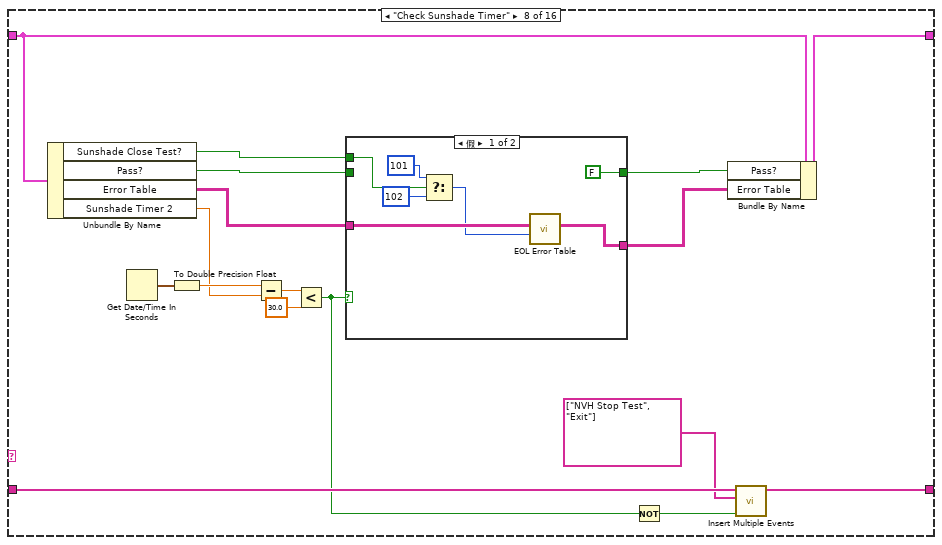
[diagram p11: hidden frame]
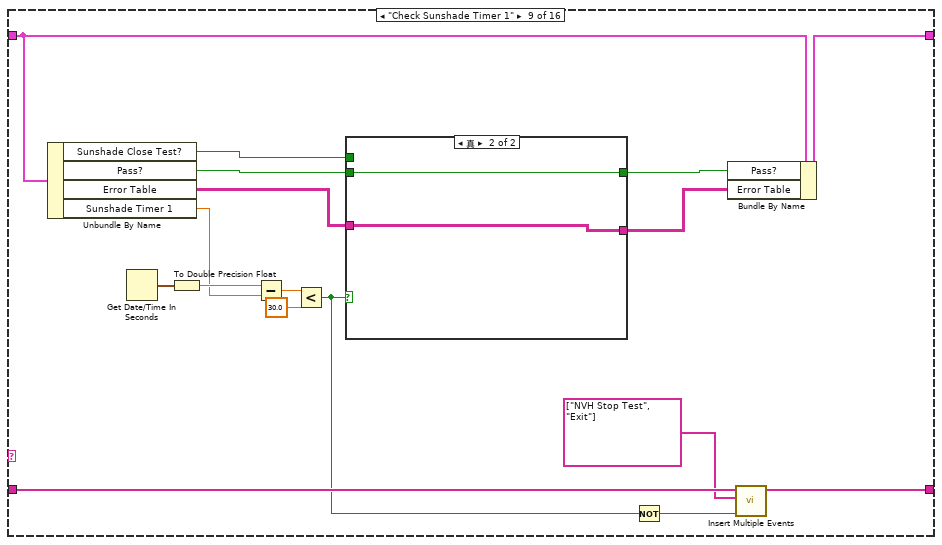
[diagram p13: hidden frame]
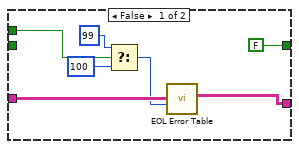
[diagram p14: hidden frame]
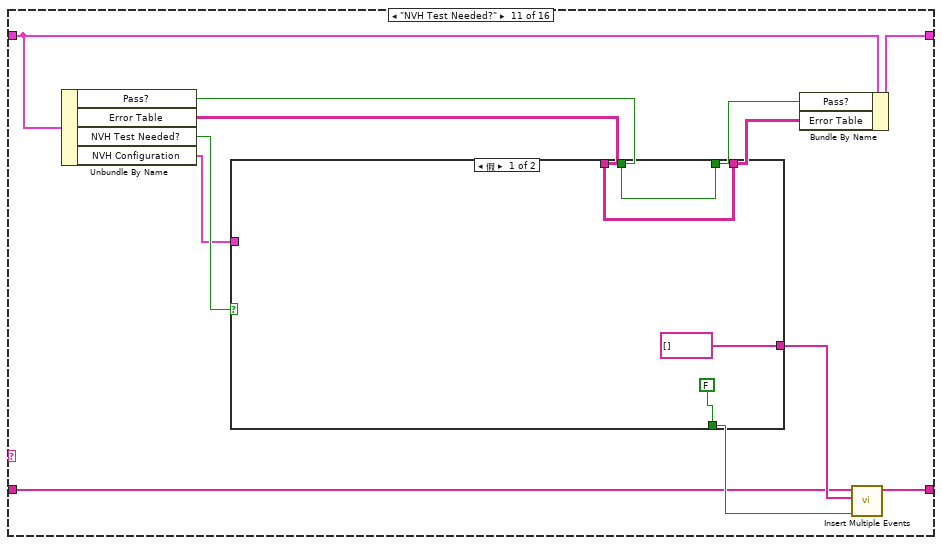
[diagram p15: hidden frame]
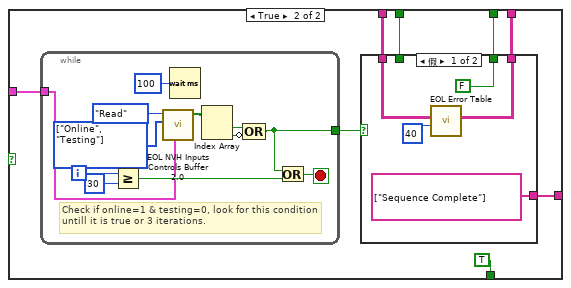
[diagram p16: hidden frame]
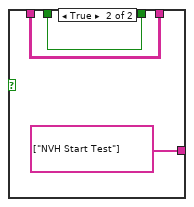
[diagram p17: hidden frame]
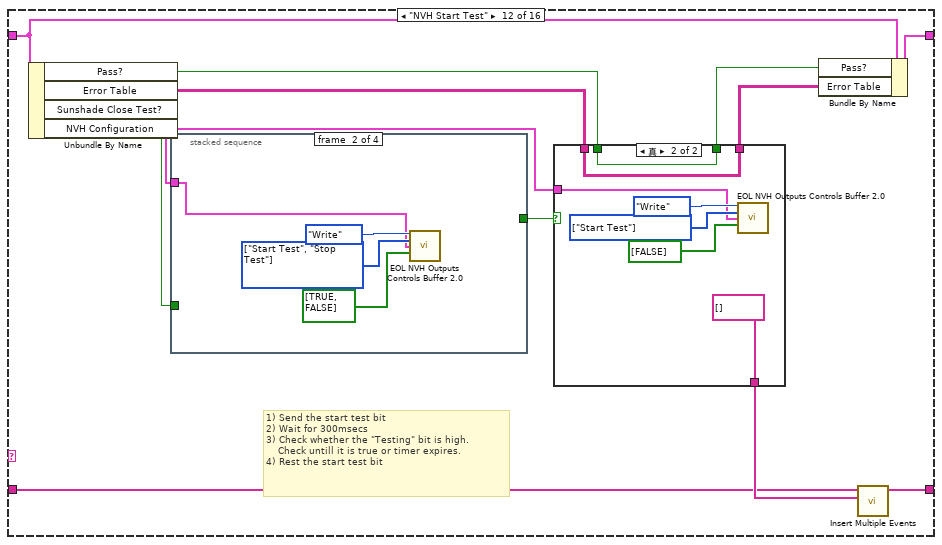
[diagram p18: hidden frame]
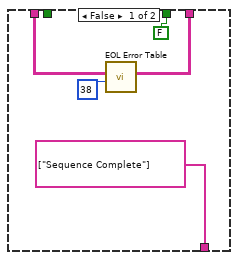
[diagram p19: hidden frame]
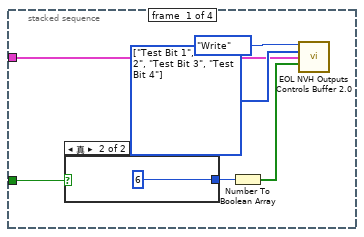
[diagram p20: hidden frame]
diagram:
  (unwired) string[] ["Open Or Close Sunshade", "NVH Test Needed?", "Check If Sunshade Moving", "Check If Sunshade Closed Or Opened", "Get Sunshade Data", "NVH Stop Test", "Calculate Sunsahde Data", "Check Sunshade Limits", "Exit"] ("event queue out")
  w12 = 0.0  # Sunshade Timer 1
  w18 = TRUE  # Pass?
  w13 = dbl[] []  # Sunshade Calculated Data
  w16 = FALSE  # NVH Test Needed?
  w14 = FALSE  # NVH Noise Test OK?
  w17 = 0.0  # Sunshade Timer 2
  w20 = dbl[] []  # Sunshade Raw Data
  n1 = Unbundle By Name("input cluster") -> ("Store Data.Error Table"=w9:string[][], "Sequence State.Step Data String"=w10:string, "Station Index"=w8:i32, "NVH Configuration"=w6:T7)  [unwired: 2 out]
  n2 = Unbundle By Name("input cluster") -> ("Config Info"=w5:T34)
  n3 = call "Config Info Get.vi"("Config Info"=w5) -> ("PLC Comms"=w3:T35)  [unwired: 7 in, 3 out]
  n4 = Unbundle By Name(w3) -> ("PLC boolean read Tags"=w2:T36, "PLC bool write Tags"=w1:T39)
  n5 = Unflatten From String(type=T1 {"Overall Min"=0.0, "Overall Max"=0.0, "Avg Min"=0.0, "Avg Max"=0.0, "Truncation Start"=0.0, "Truncation End"=0.0, "Variance"=0.0, "Check Noise"=TRUE} ("Sun Shade Close Force"), binary string=w10) -> (value=w7:T1)  [unwired: 3 in, 2 out]
  "ss servo limits" <- w7
  n6 = Bundle("Sunshade Raw Data"=w20, "Sun Shade Close Force"=w7, "Pass?"=w18, "Error Table"=w9, "Sunshade Timer 2"=w17, "NVH Test Needed?"=w16, "Sunshade Close Test?"="Sunshade Close Test?", "NVH Noise Test OK?"=w14, "Sunshade Calculated Data"=w13, "Sunshade Timer 1"=w12, "Station Index"=w8, "PLC boolean read Tags"=w2, "PLC bool write Tags"=w1, "NVH Configuration"=w6) -> (w19:T42)  [unwired: 1 in]
  n7 = while {
    shift-right: [w30] -> _
    shift-left: string[] ["Init"] ("event queue out") -> [w26]
    shift-right: [w28] -> _
    shift-left: w19 -> [w29]
    tunnel: "input cluster" -> [w22]
    stop <- w24 continue-if-true
    n8 = call "EOL next state.vi"("Main State Cluster"=w22, "event queue in"=w26) -> ("Condition (Exit:F)"=w24:bool, "next event"=w23:string, "event queue out"=w25:string[])  [unwired: 5 in, 2 out]
    "State" <- w23
    n9 = Wait (ms)(milliseconds to wait=u32 5) -> ()  [unwired: 1 out]
    n10 = case shown="\"Get Sunshade Data\"" w23 {
      selector: w23 -> [w32 _ _ _ _ _ _ _ _ _ _ _ _ _ _ _]
      tunnel: w25 -> [w36 _ _ w55 w68 w88 w104 w115 w141 w169 w174 w220 w268 w319 w351 w368]
      tunnel: [w36 string[] ["Open Or Close Sunshade", "NVH Test Needed?", "Check If Sunshade Moving", "Check If Sunshade Closed Or Opened", "Get Sunshade Data", "NVH Stop Test", "Calculate Sunsahde Data", "Check Sunshade Limits", "Exit"] ("event queue out") string[] ["Exit"] ("event queue out") w55 w67 w87 w104 w114 w140 w169 w175 w219 w267 w318 w351 w368] -> w30
      tunnel: w29 -> [w31 w37 w42 w54 w64 w84 w108 w119 w145 w168 w177 w217 w269 w317 w357 w367]
      tunnel: [w31 w37 w43 w56 w69 w84 w107 w118 w144 w167 w176 w218 w266 w316 w356 w367] -> w28
      frame "Error", Default {
        n11 = Concatenate Strings("Sunshade Test  Entered Error State - The Intended state was - " ("string"), w32) -> (w34:string)
        n12 = One Button Dialog(message=w34, button name ("OK")="OK") -> ()  [unwired: 1 out]
      }
      frame "Init" {
      }
      frame "Abort Test" {
        n13 = Unbundle By Name(w42) -> ("Error Table"=w44:string[][])
        n14 = call "EOL Error Table.vi"("Error No."=u16 28, "Error Table In"=w44) -> ("Error Table Out"=w39:string[][])  [unwired: 8 in, 1 out]
        n15 = Bundle By Name(cluster=w42, "Pass?"=FALSE, "Error Table"=w39) -> (w43:T42)
      }
      frame "Open Or Close Sunshade" {
        n16 = Unbundle By Name(w54) -> ("Sun Shade Close Force.Check Noise"=w52:bool, "Sunshade Close Test?"=w53:bool, "PLC bool write Tags.ss servo open"=w48:T37, "PLC bool write Tags.ss servo close"=w49:T37)
        n17 = Select(t=w49, s=w53, f=w48) -> (s? t:f=w47:T37)
        n18 = call "plc write bool.vi"("value"=TRUE, "addr,tag"=w47) -> ()  [unwired: 9 in, 1 out]
        n19 = Get Date/Time In Seconds() -> (seconds since 1Jan1904=w51:timestamp)
        n20 = To Double Precision Float(number=w51) -> (double precision float=w50:dbl)
        n21 = Bundle By Name(cluster=w54, "Sunshade Raw Data"=dbl[] [] ("Sunshade Data"), "NVH Test Needed?"=w52, "Sunshade Timer 1"=w50) -> (w56:T42)
      }
      frame "Check If Sunshade Moving" {
        n22 = Unbundle By Name(w64) -> ("Station Index"=w58:i32, "Sunshade Close Test?"=w63:bool, "PLC boolean read Tags.ss servo closing"=w62:T37, "PLC boolean read Tags.ss servo opening"=w61:T37)
        n23 = Select(t=w62, s=w63, f=w61) -> (s? t:f=w60:T37)
        n24 = call "plc read bool.vi"("addr,tag"=w60) -> ("value"=w59:bool)  [unwired: 9 in, 1 out]
        n25 = Get Date/Time In Seconds() -> (seconds since 1Jan1904=w66:timestamp)
        n26 = case shown="真" w59 {
          tunnel: w58 -> [_ w73]
          frame False {
          }
          frame True {
            n27 = call "EOL All-Station AI Circular Data Buffer.vi"("station idx"=w73, "Mode"=enum16{"Initialize", "Read", "Write"}."Read") -> ("Data Read (Samp-Ro, Ch-Col)"=→"Cleared data":sgl[][])  [unwired: 9 in]
          }
        }
        n28 = To Double Precision Float(number=w66) -> (double precision float=w65:dbl)
        n29 = Bundle By Name(cluster=w64, "Sunshade Timer 2"=w65, "Sunshade Raw Data"=dbl[] [] ("Sunshade Data Array")) -> (w69:T42)
        n30 = Not(x=w59) -> (.not. x?=w71:bool)
        n31 = call "Insert Multiple Events.vi"("Insert all? (T)"=w71, "Events to Insert"=string[] ["Check Sunshade Timer 1", "Check If Sunshade Moving"], "Event queue in"=w68) -> ("Event queue out"=w67:string[])  [unwired: 4 in]
      }
      frame "Check If Sunshade Closed Or Opened" {
        n32 = Unbundle By Name(w84) -> ("Sunshade Close Test?"=w83:bool, "PLC boolean read Tags.ss servo at close"=w82:T37, "PLC boolean read Tags.ss servo at open"=w81:T37, "PLC bool write Tags.ss servo close"=w80:T37, "PLC bool write Tags.ss servo open"=w79:T37)
        n33 = Select(t=w82, s=w83, f=w81) -> (s? t:f=w78:T37)
        n34 = call "plc read bool.vi"("addr,tag"=w78) -> ("error out"=w76:errorcluster, "value"=w77:bool)  [unwired: 9 in]
        n35 = case shown="真" w77 {
          tunnel: w83 -> [_ w96]
          tunnel: w80 -> [_ w95]
          tunnel: w79 -> [_ w94]
          tunnel: w76 -> [w89 w91]
          tunnel: [w89 w90] -> _
          frame False {
          }
          frame True {
            n36 = Select(t=w95, s=w96, f=w94) -> (s? t:f=w93:T37)
            n37 = call "plc write bool.vi"("error in"=w91, "value"=FALSE, "addr,tag"=w93) -> ("error out"=w90:errorcluster)  [unwired: 8 in]
          }
        }
        n38 = Not(x=w77) -> (.not. x?=w86:bool)
        n39 = call "Insert Multiple Events.vi"("Insert all? (T)"=w86, "Events to Insert"=string[] ["Check Sunshade Timer", "Check If Sunshade Closed Or Opened"], "Event queue in"=w88) -> ("Event queue out"=w87:string[])  [unwired: 4 in]
      }
      frame "Calculate Sunsahde Data" {
        n40 = Unbundle By Name(w108) -> ("Sunshade Raw Data"=w109:dbl[], "Sun Shade Close Force.Truncation Start"=w106:dbl, "Sun Shade Close Force.Truncation End"=w105:dbl)
        n41 = Multiply(x=w109, y="scaling factor") -> (x*y=w102:dbl[])
        n42 = Absolute Value(x=w102) -> (abs(x)=w98:dbl[])
        "Current Out" <- w98
        n43 = To Long Integer(number=w106) -> (32bit integer=w101:i32)
        n44 = To Long Integer(number=w105) -> (32bit integer=w100:i32)
        n45 = call "EOL Calculate Sunshade Data.vi"("Truncation End"=w100, "Truncation Start"=w101, "Array Data"=w98) -> ("Current Out"=→"Current Out New":dbl[], "Sunshade Data"=w99:dbl[])  [unwired: 7 in]
        n46 = Bundle By Name(cluster=w108, "Sunshade Raw Data"=w98, "Sunshade Calculated Data"=w99) -> (w107:T42)
      }
      frame "Check Sunshade Timer" {
        n47 = Unbundle By Name(w119) -> ("Sunshade Close Test?"=w110:bool, "Pass?"=w120:bool, "Error Table"=w121:string[][], "Sunshade Timer 2"=w122:dbl)
        n48 = Get Date/Time In Seconds() -> (seconds since 1Jan1904=w126:timestamp)
        n49 = To Double Precision Float(number=w126) -> (double precision float=w125:dbl)
        n50 = Subtract(x=w125, y=w122) -> (x-y=w124:dbl)
        n51 = Less?(x=w124, y=30.0) -> (x < y?=w112:bool)
        n52 = case shown="假" w112 {
          tunnel: w120 -> [_ w134]
          tunnel: w121 -> [w129 w135]
          tunnel: [w128 w135] -> w116
          tunnel: [FALSE ("Pass?") w134] -> w117
          tunnel: w110 -> [w132 _]
          frame False {
            n53 = Select(t=u16 101 ("Error No."), s=w132, f=u16 102) -> (s? t:f=w127:u16)
            n54 = call "EOL Error Table.vi"("Error No."=w127, "Error Table In"=w129) -> ("Error Table Out"=w128:string[][])  [unwired: 8 in, 1 out]
          }
          frame True {
          }
        }
        n55 = Not(x=w112) -> (.not. x?=w111:bool)
        n56 = Bundle By Name(cluster=w119, "Pass?"=w117, "Error Table"=w116) -> (w118:T42)
        n57 = call "Insert Multiple Events.vi"("Insert all? (T)"=w111, "Events to Insert"=string[] ["NVH Stop Test", "Exit"], "Event queue in"=w115) -> ("Event queue out"=w114:string[])  [unwired: 4 in]
      }
      frame "Check Sunshade Timer 1" {
        n58 = Unbundle By Name(w145) -> ("Sunshade Close Test?"=w136:bool, "Pass?"=w146:bool, "Error Table"=w147:string[][], "Sunshade Timer 1"=w148:dbl)
        n59 = Get Date/Time In Seconds() -> (seconds since 1Jan1904=w152:timestamp)
        n60 = To Double Precision Float(number=w152) -> (double precision float=w151:dbl)
        n61 = Subtract(x=w151, y=w148) -> (x-y=w150:dbl)
        n62 = Less?(x=w150, y=30.0) -> (x < y?=w138:bool)
        n63 = case shown="真" w138 {
          tunnel: w146 -> [_ w160]
          tunnel: w147 -> [w156 w161]
          tunnel: [w154 w161] -> w142
          tunnel: [FALSE ("Pass?") w160] -> w143
          tunnel: w136 -> [w155 _]
          frame False {
            n64 = Select(t=u16 99 ("Error No."), s=w155, f=u16 100) -> (s? t:f=w153:u16)
            n65 = call "EOL Error Table.vi"("Error No."=w153, "Error Table In"=w156) -> ("Error Table Out"=w154:string[][])  [unwired: 8 in, 1 out]
          }
          frame True {
          }
        }
        n66 = Not(x=w138) -> (.not. x?=w137:bool)
        n67 = Bundle By Name(cluster=w145, "Pass?"=w143, "Error Table"=w142) -> (w144:T42)
        n68 = call "Insert Multiple Events.vi"("Insert all? (T)"=w137, "Events to Insert"=string[] ["NVH Stop Test", "Exit"], "Event queue in"=w141) -> ("Event queue out"=w140:string[])  [unwired: 4 in]
      }
      frame "Get Sunshade Data" {
        n69 = Unbundle By Name(w168) -> ("Sunshade Raw Data"=w171:dbl[], "Station Index"=w164:i32)
        n70 = call "EOL All-Station AI Circular Data Buffer.vi"("station idx"=w164, "Mode"=enum16{"Initialize", "Read", "Write"}."Read") -> ("Data Read (Samp-Ro, Ch-Col)"=w165:sgl[][])  [unwired: 9 in]
        n71 = Index Array(array=w165, index (col)=EOL_Analog_Input_Control."SW PS  Volage" ("Analog Control")) -> (element=w162:sgl[])  [unwired: 1 in]
        n72 = Build Array (concatenate)(w171, w162) -> (w170:dbl[])
        n73 = Bundle By Name(cluster=w168, "Sunshade Raw Data"=w170) -> (w167:T42)
      }
      frame "NVH Test Needed?" {
        n74 = Unbundle By Name(w177) -> ("Pass?"=w182:bool, "Error Table"=w183:string[][], "NVH Test Needed?"=w173:bool, "NVH Configuration"=w172:T7)
        n75 = case shown="假" w173 {
          tunnel: w183 -> [w187 w194]
          tunnel: [w187 w193] -> w180
          tunnel: w182 -> [w186 w191]
          tunnel: [w186 w192] -> w181
          tunnel: [string[] [] ("event queue out") w190] -> w179
          tunnel: [FALSE TRUE] -> w178
          tunnel: w172 -> [_ w188]
          frame False {
          }
          frame True {
            n76 = while {
              tunnel: [w206] -> w195
              tunnel: w188 -> [w204]
              i -> [w215]
              stop <- w212 stop-if-true
              w210 = T45[] [enum."Online", enum."Testing"] items=["Online", "Pass", "Fail", "Testing", "Ready for Model", "Error Bit 1", "Error Bit 2", "Error Bit 3", "Failure Bit 1", "Failure Bit 2", "Failure Bit 3", "Failure Bit 4", "Echo Bit 1", "Echo Bit 2", "Echo Bit 3", "Echo Bit 4", "Serial Number Read Ok", "Ready for Serrial Number"] ("Digital Inputs Array")
              # "Check if online=1 & testing=0, look for this condition\nuntill it is true or 3 iterations."
              n77 = Greater Or Equal?(x=w215, y=30) -> (x >= y?=w213:bool)
              n78 = call "EOL NVH Inputs Controls Buffer 2.0.vi"("NVH Configuration"=w204, "NVHK Inputs Control"=w210, "Mode"=NVH_Mode_Control_2.0."Read") -> ("NVH Inputs Out"=w207:bool[])  [unwired: 4 in, 4 out]
              n79 = Wait (ms)(milliseconds to wait=u32 100) -> ()  [unwired: 1 out]
              n80 = Index Array(array=w207) -> (element #1=w209:bool, element #2=w208:bool)  [unwired: 2 in]
              n81 = Compound Arithmetic op=OR(w209, invert w208) -> (w206:bool)
              n82 = Or(x=w206, y=w213) -> (x .or. y?=w212:bool)
            }
            n83 = case shown="假" w195 {
              tunnel: w194 -> [w200 w202]
              tunnel: [w197 w202] -> w193
              tunnel: [FALSE ("Pass?") w203] -> w192
              tunnel: w191 -> [_ w203]
              tunnel: [string[] ["Sequence Complete"] ("event queue out") string[] ["NVH Start Test"] ("event queue out")] -> w190
              frame False {
                n84 = call "EOL Error Table.vi"("Error No."=u16 40, "Error Table In"=w200) -> ("Error Table Out"=w197:string[][])  [unwired: 8 in, 1 out]
              }
              frame True {
              }
            }
          }
        }
        n85 = Bundle By Name(cluster=w177, "Pass?"=w181, "Error Table"=w180) -> (w176:T42)
        n86 = call "Insert Multiple Events.vi"("Insert all? (T)"=w178, "Events to Insert"=w179, "Event queue in"=w174) -> ("Event queue out"=w175:string[])  [unwired: 1 in, 3 out]
      }
      frame "NVH Start Test" {
        # "1) Send the start test bit\n2) Wait for 300msecs\n3) Check whether the \"Testing\" bit is high.\n    Check untill it is true or timer expires.\n4) Rest the start test bit"
        n87 = Unbundle By Name(w217) -> ("Pass?"=w224:bool, "Error Table"=w225:string[][], "Sunshade Close Test?"=w227:bool, "NVH Configuration"=w216:T7)
        n88 = stacked-sequence {
          tunnel: w227 -> [w241 _ _ _]
          tunnel: [_ _ _ w254] -> w221
          tunnel: w216 -> [w240 w248 _ w253]
          frame #0 {
            w244 = T46[] [enum."Test Bit 1", enum."Test Bit 2", enum."Test Bit 3", enum."Test Bit 4"] items=["Restart IRQ", "Abort Test IRQ", "Read Model", "Start Test", "Stop Test", "End of Test IRQ", "Test Bit 1", "Test Bit 2", "Test Bit 3", "Test Bit 4", "Model Bit 1", "Model Bit 2", "Model Bit 3", "Model Bit 4", "Manual Restart IRQ"] ("B&K Outputs Control")
            n89 = case shown="真" w241 {
              tunnel: [u8 5 u8 6] -> w243
              frame False {
              }
              frame True {
              }
            }
            n90 = Number To Boolean Array(number=w243) -> (Boolean array=w242:bool[])
            n91 = call "EOL NVH Outputs Controls Buffer 2.0.vi"("Mode"=NVH_Mode_Control_2.0."Write", "NVH Outputs Control"=w244, "NVH Configuration"=w240, "NVH Outputs"=w242) -> ()  [unwired: 6 in, 6 out]
          }
          frame #1 {
            w250 = T46[] [enum."Start Test", enum."Stop Test"] items=["Restart IRQ", "Abort Test IRQ", "Read Model", "Start Test", "Stop Test", "End of Test IRQ", "Test Bit 1", "Test Bit 2", "Test Bit 3", "Test Bit 4", "Model Bit 1", "Model Bit 2", "Model Bit 3", "Model Bit 4", "Manual Restart IRQ"] ("B&K Outputs Control")
            n92 = call "EOL NVH Outputs Controls Buffer 2.0.vi"("Mode"=NVH_Mode_Control_2.0."Write", "NVH Outputs Control"=w250, "NVH Configuration"=w248, "NVH Outputs"=bool[] [TRUE, FALSE]) -> ()  [unwired: 6 in, 6 out]
          }
          frame #2 {
            n93 = Wait (ms)(milliseconds to wait=u32 300 ("START TEST STEP B&K")) -> ()  [unwired: 1 out]
          }
          frame #3 {
            n94 = while {
              tunnel: [w257] -> w254
              tunnel: w253 -> [w255]
              i -> [w263]
              stop <- w260 stop-if-true
              w258 = T45[] [enum."Testing"] items=["Online", "Pass", "Fail", "Testing", "Ready for Model", "Error Bit 1", "Error Bit 2", "Error Bit 3", "Failure Bit 1", "Failure Bit 2", "Failure Bit 3", "Failure Bit 4", "Echo Bit 1", "Echo Bit 2", "Echo Bit 3", "Echo Bit 4", "Serial Number Read Ok", "Ready for Serrial Number"] ("Digital Inputs Array")
              # "Check if testing=1, look for this condition\nuntill it is true or 5 seconds expire."
              n95 = Greater Or Equal?(x=w263, y=50) -> (x >= y?=w261:bool)
              n96 = call "EOL NVH Inputs Controls Buffer 2.0.vi"("NVH Configuration"=w255, "NVHK Inputs Control"=w258, "Mode"=NVH_Mode_Control_2.0."Read") -> ("NVH Single Input"=w257:bool)  [unwired: 4 in, 4 out]
              n97 = Or(x=w257, y=w261) -> (x .or. y?=w260:bool)
              n98 = Wait (ms)(milliseconds to wait=u32 100) -> ()  [unwired: 1 out]
            }
          }
        }
        n99 = case shown="真" w221 {
          tunnel: [string[] ["Sequence Complete"] ("event queue out") string[] [] ("event queue out")] -> w226
          tunnel: w225 -> [w231 w237]
          tunnel: w224 -> [_ w238]
          tunnel: [FALSE ("Pass?") w238] -> w223
          tunnel: [w229 w237] -> w222
          tunnel: w216 -> [_ w233]
          frame False {
            n100 = call "EOL Error Table.vi"("Error No."=u16 38, "Error Table In"=w231) -> ("Error Table Out"=w229:string[][])  [unwired: 8 in, 1 out]
          }
          frame True {
            w235 = T46[] [enum."Start Test"] items=["Restart IRQ", "Abort Test IRQ", "Read Model", "Start Test", "Stop Test", "End of Test IRQ", "Test Bit 1", "Test Bit 2", "Test Bit 3", "Test Bit 4", "Model Bit 1", "Model Bit 2", "Model Bit 3", "Model Bit 4", "Manual Restart IRQ"] ("B&K Outputs Control")
            n101 = call "EOL NVH Outputs Controls Buffer 2.0.vi"("Mode"=NVH_Mode_Control_2.0."Write", "NVH Outputs Control"=w235, "NVH Configuration"=w233, "NVH Outputs"=bool[] [FALSE]) -> ()  [unwired: 6 in, 6 out]
          }
        }
        n102 = Bundle By Name(cluster=w217, "Pass?"=w223, "Error Table"=w222) -> (w218:T42)
        n103 = call "Insert Multiple Events.vi"("Events to Insert"=w226, "Event queue in"=w220) -> ("Event queue out"=w219:string[])  [unwired: 2 in, 3 out]
      }
      frame "NVH Stop Test" {
        # "1) Send Stop Test bit only when the NVH system is running\n2) Send the stop test bit\n3) Wait for 300msecs\n4) Check whether the \"Testing\" bit is low.   Check untill it is false or timer expires.\n5) ResEt the stop test bit"
        n104 = Unbundle By Name(w269) -> ("Pass?"=w272:bool, "Error Table"=w273:string[][], "NVH Test Needed?"=w265:bool, "NVH Configuration"=w264:T7)
        n105 = case shown="假" w265 {
          tunnel: [string[] [] ("event queue out") w283] -> w274
          tunnel: w273 -> [w275 w282]
          tunnel: w272 -> [w276 w281]
          tunnel: [w276 w280] -> w271
          tunnel: [w275 w279] -> w270
          tunnel: w264 -> [_ w278]
          frame False {
          }
          frame True {
            n106 = stacked-sequence {
              tunnel: [_ _ w299 _] -> w284
              tunnel: w278 -> [w293 _ w298 w309]
              frame #0 {
                w295 = T46[] [enum."Stop Test", enum."Start Test"] items=["Restart IRQ", "Abort Test IRQ", "Read Model", "Start Test", "Stop Test", "End of Test IRQ", "Test Bit 1", "Test Bit 2", "Test Bit 3", "Test Bit 4", "Model Bit 1", "Model Bit 2", "Model Bit 3", "Model Bit 4", "Manual Restart IRQ"] ("B&K Outputs Control")
                n107 = call "EOL NVH Outputs Controls Buffer 2.0.vi"("Mode"=NVH_Mode_Control_2.0."Write", "NVH Outputs Control"=w295, "NVH Configuration"=w293, "NVH Outputs"=bool[] [TRUE, FALSE]) -> ()  [unwired: 6 in, 6 out]
              }
              frame #1 {
                n108 = Wait (ms)(milliseconds to wait=u32 100 ("START TEST STEP B&K")) -> ()  [unwired: 1 out]
              }
              frame #2 {
                n109 = while {
                  tunnel: [w302] -> w299
                  tunnel: w298 -> [w300]
                  i -> [w308]
                  stop <- w305 stop-if-true
                  w303 = T45[] [enum."Testing"] items=["Online", "Pass", "Fail", "Testing", "Ready for Model", "Error Bit 1", "Error Bit 2", "Error Bit 3", "Failure Bit 1", "Failure Bit 2", "Failure Bit 3", "Failure Bit 4", "Echo Bit 1", "Echo Bit 2", "Echo Bit 3", "Echo Bit 4", "Serial Number Read Ok", "Ready for Serrial Number"] ("Digital Inputs Array")
                  # "Check if testing=0, look for this condition\nuntill it is true or 15 seconds expire."
                  n110 = Greater Or Equal?(x=w308, y=150) -> (x >= y?=w306:bool)
                  n111 = call "EOL NVH Inputs Controls Buffer 2.0.vi"("NVH Configuration"=w300, "NVHK Inputs Control"=w303, "Mode"=NVH_Mode_Control_2.0."Read") -> ("NVH Single Input"=w302:bool)  [unwired: 4 in, 4 out]
                  n112 = Compound Arithmetic op=OR(invert w302, w306) -> (w305:bool)
                  n113 = Wait (ms)(milliseconds to wait=u32 100) -> ()  [unwired: 1 out]
                }
              }
              frame #3 {
                w311 = T46[] [enum."Stop Test"] items=["Restart IRQ", "Abort Test IRQ", "Read Model", "Start Test", "Stop Test", "End of Test IRQ", "Test Bit 1", "Test Bit 2", "Test Bit 3", "Test Bit 4", "Model Bit 1", "Model Bit 2", "Model Bit 3", "Model Bit 4", "Manual Restart IRQ"] ("B&K Outputs Control")
                n114 = call "EOL NVH Outputs Controls Buffer 2.0.vi"("Mode"=NVH_Mode_Control_2.0."Write", "NVH Outputs Control"=w311, "NVH Configuration"=w309, "NVH Outputs"=bool[] [FALSE]) -> ()  [unwired: 6 in, 6 out]
              }
            }
            n115 = case shown="真" w284 {
              tunnel: [string[] ["NVH Check Error"] ("event queue out") string[] ["Sequence Complete"] ("event queue out")] -> w283
              tunnel: w282 -> [w286 w291]
              tunnel: w281 -> [w287 _]
              tunnel: [w287 FALSE ("Pass?")] -> w280
              tunnel: [w286 w288] -> w279
              frame False {
              }
              frame True {
                n116 = call "EOL Error Table.vi"("Error No."=u16 39, "Error Table In"=w291) -> ("Error Table Out"=w288:string[][])  [unwired: 8 in, 1 out]
              }
            }
          }
        }
        n117 = Bundle By Name(cluster=w269, "Pass?"=w271, "Error Table"=w270) -> (w266:T42)
        n118 = call "Insert Multiple Events.vi"("Events to Insert"=w274, "Event queue in"=w268) -> ("Event queue out"=w267:string[])  [unwired: 2 in, 3 out]
      }
      frame "NVH Check Error" {
        w326 = T45[] [enum."Pass", enum."Fail"] items=["Online", "Pass", "Fail", "Testing", "Ready for Model", "Error Bit 1", "Error Bit 2", "Error Bit 3", "Failure Bit 1", "Failure Bit 2", "Failure Bit 3", "Failure Bit 4", "Echo Bit 1", "Echo Bit 2", "Echo Bit 3", "Echo Bit 4", "Serial Number Read Ok", "Ready for Serrial Number"] ("Digital Inputs Array")
        # "1) Reset the Stop Bit\n2) Check if there is an failure. If there are then \n     report the failure\n3) Check if there are any errors with the system (This needs to be added in later"
        n119 = Unbundle By Name(w317) -> ("Pass?"=w314:bool, "Error Table"=w330:string[][], "Sun Shade Close Force.Check Noise"=w323:bool, "NVH Configuration"=w313:T7)
        n120 = call "EOL NVH Inputs Controls Buffer 2.0.vi"("NVH Configuration"=w313, "NVHK Inputs Control"=w326, "Mode"=NVH_Mode_Control_2.0."Read") -> ("Error out"=w320:string[][], "NVH Inputs Out"=w329:bool[])  [unwired: 4 in, 3 out]
        n121 = Boolean Array To Number(Boolean array=w329) -> (number=w328:u32)
        n122 = stacked-sequence {
          tunnel: w330 -> [_ w340]
          tunnel: w328 -> [_ w339]
          tunnel: [_ w338] -> w327
          tunnel: [_ w337] -> w315
          tunnel: w323 -> [_ w336]
          tunnel: w320 -> [_ w335]
          tunnel: w313 -> [w331 _]
          frame #0 {
            w333 = T46[] [enum."Stop Test"] items=["Restart IRQ", "Abort Test IRQ", "Read Model", "Start Test", "Stop Test", "End of Test IRQ", "Test Bit 1", "Test Bit 2", "Test Bit 3", "Test Bit 4", "Model Bit 1", "Model Bit 2", "Model Bit 3", "Model Bit 4", "Manual Restart IRQ"] ("B&K Outputs Control")
            n123 = call "EOL NVH Outputs Controls Buffer 2.0.vi"("Mode"=NVH_Mode_Control_2.0."Write", "NVH Outputs Control"=w333, "NVH Configuration"=w331, "NVH Outputs"=bool[] [FALSE]) -> ()  [unwired: 6 in, 6 out]
          }
          frame #1 {
            n124 = case shown="2" w339 {
              tunnel: w340 -> [w342 w346]
              tunnel: [w342 w344] -> w338
              tunnel: [TRUE w343] -> w337
              tunnel: w336 -> [_ w349]
              tunnel: w335 -> [_ w345]
              frame 0, Default {
              }
              frame 2 {
                n125 = Select(t=FALSE ("Pass/Fail"), s=w349, f=TRUE) -> (s? t:f=w343:bool)
                n126 = Build Array (concatenate)(w346, w345) -> (w344:string[][])
              }
            }
          }
        }
        n127 = And(x=w314, y=w315) -> (x .and. y?=w322:bool)
        n128 = Not(x=w315) -> (.not. x?=w324:bool)
        n129 = Bundle By Name(cluster=w317, "Pass?"=w322, "Error Table"=w327, "NVH Noise Test OK?"=w315) -> (w316:T42)
        n130 = call "Insert Multiple Events.vi"("Insert all? (T)"=w324, "Events to Insert"=string[] ["Sequence Complete"], "Event queue in"=w319) -> ("Event queue out"=w318:string[])  [unwired: 1 in, 3 out]
      }
      frame "Check Sunshade Limits" {
        n131 = Unbundle By Name(w357) -> ("Sunshade Calculated Data"=w352:dbl[], "Sun Shade Close Force"=w353:T1, "Sunshade Close Test?"=w359:bool, "Error Table"=w354:string[][])
        n132 = call "EOL Check Sunshade Limits.vi"("Error Table"=w354, "Sunshade Close?"=w359, "Sun Shade Limits"=w353, "Sunshade Calculated Data"=w352) -> ("Error Table 2"=w355:string[][], "All Sunshade Data and Limits"=w350:dbl[], "Pass?"=w358:bool)  [unwired: 5 in]
        n133 = Bundle By Name(cluster=w357, "Pass?"=w358, "Sunshade Calculated Data"=w350, "Error Table"=w355) -> (w356:T42)
      }
      frame "Exit" {
        n134 = Unbundle By Name(w367) -> ("Pass?"=→"Pass? Out":bool, "Error Table"=→"Error Table Out":string[][], "Sunshade Calculated Data"=→"Sunshade Calculated Data":dbl[], "Sunshade Raw Data"=→"Sunshade Raw Data":dbl[], "PLC bool write Tags.ss servo open"=w362:T37, "PLC bool write Tags.ss servo close"=w361:T37)
        n135 = Build Array(w362, w361) -> (w360:T37[])
        n136 = for {
          tunnel: w360 -> [w369] mode=indexing
          n137 = call "plc write bool.vi"("value"=FALSE, "addr,tag"=w369) -> ()  [unwired: 9 in, 1 out]
        }
      }
    }
  }
